vi "FeedbackDecode_InWindowMDim.vi"(4 "Jitter":dbl, 5 "Radius":dbl=0.1, 6 "Targ":dbl[](array[numeric])=[0.0, 0.0, 0.0, 0.0, 0.0, 0.0, 0.0, 0.0, 0.0, 0.0], 7 "Pos":dbl[](array[numeric])=[0.0, 0.0, 0.0, 0.0, 0.0, 0.0, 0.0, 0.0, 0.0, 0.0]) -> (0 "Status":enum16{"In", "Out"}(ring)=enum."Out", 1 "TargStatus":i16[](array[numeric]), 2 "TargDist":dbl[](array[numeric]), 3 "TargStim":i16[](array[numeric]))   [LabVIEW 2020]
panel:
  # "All coords normalized from 0 to 1. Up to 10 dimensions can be used."
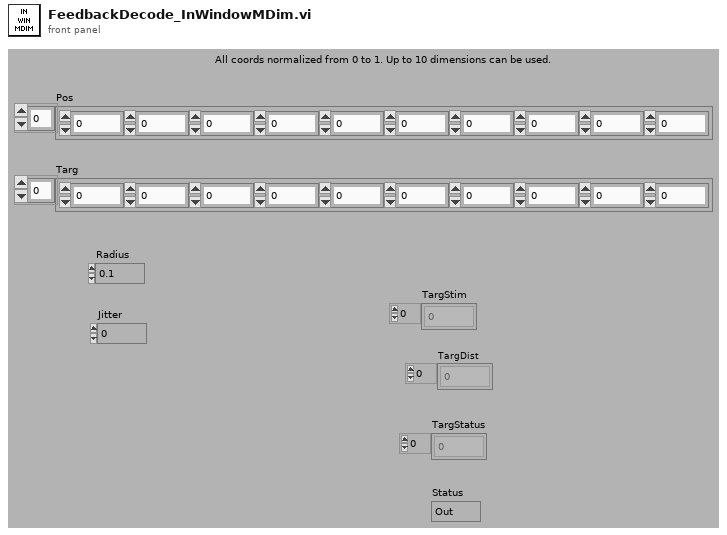
[diagram p1: front panel]
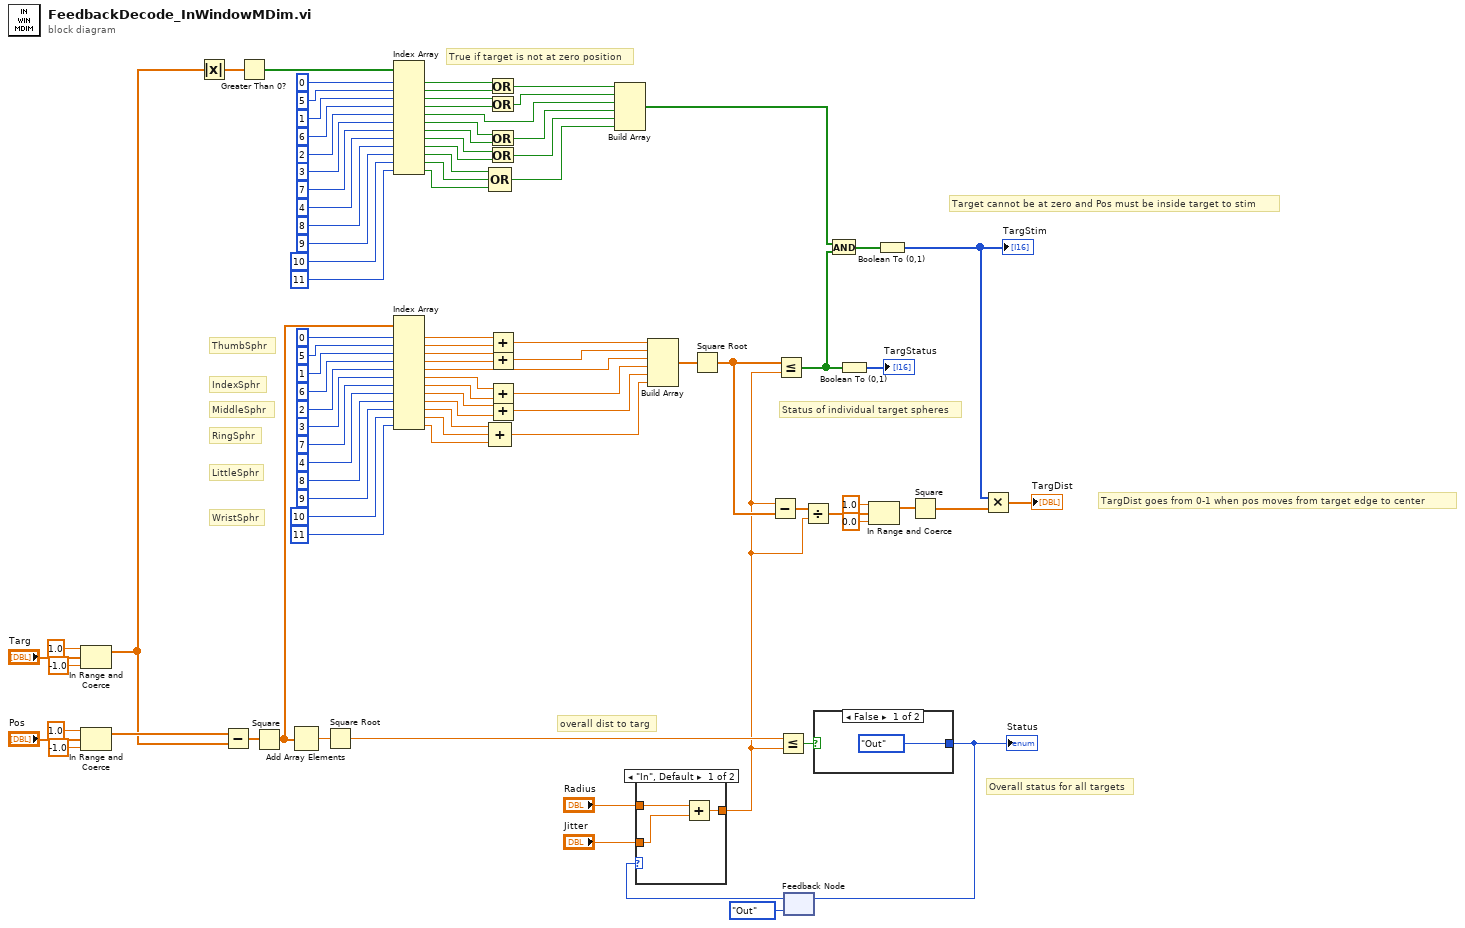
[diagram p0: block diagram]
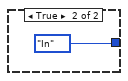
[diagram p3: hidden frame]
diagram:
  # "True if target is not at zero position"
  # "overall dist to targ"
  # "Target cannot be at zero and Pos must be inside target to stim"
  # "Overall status for all targets"
  # "Status of individual target spheres"
  # "WristSphr"
  # "LittleSphr"
  # "RingSphr"
  # "MiddleSphr"
  # "IndexSphr"
  # "ThumbSphr"
  # "TargDist goes from 0-1 when pos moves from target edge to center"
  n1 = In Range and Coerce(upper limit=1.0, x="Targ", lower limit=-1.0) -> (coerced(x)=w1:dbl[])  [unwired: 1 out]
  n2 = In Range and Coerce(upper limit=1.0, x="Pos", lower limit=-1.0) -> (coerced(x)=w83:dbl[])  [unwired: 1 out]
  n3 = Absolute Value(x=w1) -> (abs(x)=w33:dbl[])
  n4 = Subtract(x=w83, y=w1) -> (x-y=w90:dbl[])
  n5 = Greater Than 0?(x=w33) -> (x > 0?=w32:bool[])
  n6 = Square(x=w90) -> (x^2=w81:dbl[])
  n7 = Add Array Elements(numeric array=w81) -> (sum=w89:dbl)
  n8 = Square Root(x=w89) -> (sqrt(x)=w82:dbl)
  n9 = Index Array(array=w32, index #1=0 ("index"), index #2=5 ("index"), index #3=1 ("index"), index #4=6 ("index"), index #5=2 ("index"), index #6=3 ("index"), index #7=7 ("index"), index #8=4 ("index"), index #9=8 ("index"), index #10=9 ("index"), index #11=10 ("index"), index #12=11 ("index")) -> (element #1=w36:bool, element #2=w37:bool, element #3=w48:bool, element #4=w49:bool, element #5=w29:bool, element #6=w50:bool, element #7=w51:bool, element #8=w52:bool, element #9=w53:bool, element #10=w54:bool, element #11=w55:bool, element #12=w56:bool)
  n10 = Index Array(array=w81, index #1=0 ("index"), index #2=5 ("index"), index #3=1 ("index"), index #4=6 ("index"), index #5=2 ("index"), index #6=3 ("index"), index #7=7 ("index"), index #8=4 ("index"), index #9=8 ("index"), index #10=9 ("index"), index #11=10 ("index"), index #12=11 ("index")) -> (element #1=w78:dbl, element #2=w77:dbl, element #3=w66:dbl, element #4=w65:dbl, element #5=w13:dbl, element #6=w64:dbl, element #7=w63:dbl, element #8=w62:dbl, element #9=w61:dbl, element #10=w60:dbl, element #11=w59:dbl, element #12=w58:dbl)
  n11 = Or(x=w36, y=w37) -> (x .or. y?=w31:bool)
  n12 = Or(x=w48, y=w49) -> (x .or. y?=w30:bool)
  n13 = Or(x=w50, y=w51) -> (x .or. y?=w28:bool)
  n14 = Or(x=w52, y=w53) -> (x .or. y?=w27:bool)
  n15 = Add(x=w78, y=w77) -> (x+y=w15:dbl)
  n16 = Add(x=w66, y=w65) -> (x+y=w14:dbl)
  n17 = Add(x=w64, y=w63) -> (x+y=w12:dbl)
  n18 = Add(x=w62, y=w61) -> (x+y=w11:dbl)
  n19 = Compound Arithmetic op=OR(w54, w55, w56) -> (w26:bool)
  n20 = Compound Arithmetic op=ADD(w60, w59, w58) -> (w10:dbl)
  n21 = Build Array(w31, w30, w29, w28, w27, w26) -> (w25:bool[])
  n22 = Build Array(w15, w14, w13, w12, w11, w10) -> (w17:dbl[])
  n23 = Square Root(x=w17) -> (sqrt(x)=w9:dbl[])
  n24 = feedback #1(enum16{"In", "Out"}."Out" ("Fix.Status")) -> (w92:enum16{"In", "Out"})
  n25 = case shown="\"In\", Default" w92 {
    tunnel: [w96 w97] -> w8
    tunnel: "Radius" -> [w95 w97]
    tunnel: "Jitter" -> [w94 _]
    frame "In", Default {
      n26 = Add(x=w95, y=w94) -> (x+y=w96:dbl)
    }
    frame "Out" {
    }
  }
  n27 = Subtract(x=w8, y=w9) -> (x-y=w19:dbl[])
  n28 = Less Or Equal?(x=w9, y=w8) -> (x <= y?=w16:bool[])
  n29 = Less Or Equal?(x=w82, y=w8) -> (x <= y?=w93:bool)
  n30 = Divide(x=w19, y=w8) -> (x/y=w22:dbl[])
  n31 = case shown="False" w93 {
    tunnel: [enum16{"In", "Out"}."Out" ("Fix.Status") enum16{"In", "Out"}."In" ("Fix.Status")] -> w91
    frame False {
    }
    frame True {
    }
  }
  "Status" <- w91
  n32 = feedback-in #1(w91) -> ()
  n33 = And(x=w25, y=w16) -> (x .and. y?=w24:bool[])
  n34 = Boolean To (0,1)(Boolean=w16) -> (0, 1=→"TargStatus":i16[])
  n35 = In Range and Coerce(upper limit=1.0, x=w22, lower limit=0.0) -> (coerced(x)=w23:dbl[])  [unwired: 1 out]
  n36 = Boolean To (0,1)(Boolean=w24) -> (0, 1=w7:i16[])
  "TargStim" <- w7
  n37 = Square(x=w23) -> (x^2=w6:dbl[])
  n38 = Multiply(x=w7, y=w6) -> (x*y=→"TargDist":dbl[])
